vi "Filter For Replacement Terms.vi"(11 "SubVI in":refnum<vi>) -> (3 "Terms[]":refnum<vi>[](array[refnum]))   [LabVIEW 2020, in "Message Maker.lvlib"]
uses:
  Message Maker.lvlib
  <vilib>/Utility/Data Type/NI_Data Type.lvlib
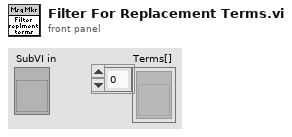
[diagram p1: front panel]
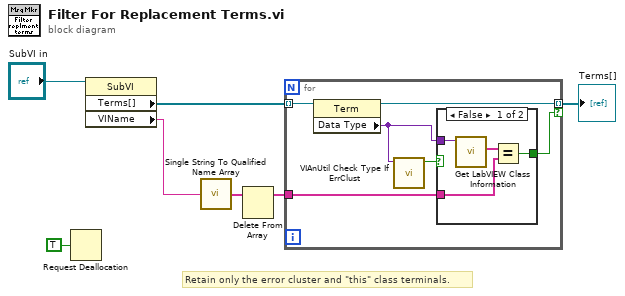
[diagram p0: block diagram]
diagram:
  # "Retain only the error cluster and \"this\" class terminals."
  n1 = Request Deallocation(TRUE ("flag")) -> ()
  n2 = property class="SubVI"(reference="SubVI in") -> ("Terms[]"=w6:refnum<vi>[], "VIName"=w5:string)  [unwired: 1 in, 2 out]
  n3 = call <vilib>:"Single String To Qualified Name Array.vi"("Fully Qualified String"=w5) -> ("Fully Qualified Array"=w4:string[])
  n4 = Delete From Array(array=w4) -> (array with subset deleted=w2:string[])  [unwired: 2 in, 1 out]
  n5 = for {
    tunnel: w6 -> [w13] mode=indexing
    tunnel: [w11] -> w3 mode=indexing if=w10
    tunnel: w2 -> [w8]
    n6 = property class="Term"(reference=w13) -> (reference out=w11:refnum<vi>, "Data Type"=w9:variant)  [unwired: 1 in, 1 out]
    n7 = call <vilib>:"VIAnUtil Check Type If ErrClust.vi"("Data In"=w9) -> ("IsErrClust?"=w12:bool)  [unwired: 9 in, 1 out]
    n8 = case shown="False" w12 {
      selector: w12 -> [_ w18]
      tunnel: [w14 w18] -> w10
      tunnel: w9 -> [w17 _]
      tunnel: w8 -> [w15 _]
      frame False {
        n9 = call <vilib>:"Get LabVIEW Class Information.vi"("variant"=w17) -> ("qualified LabVIEW class name"=w16:string[])  [unwired: 8 in, 2 out]
        n10 = Equal?(x=w16, y=w15) -> (x = y?=w14:bool)
      }
      frame True {
      }
    }
  }
  "Terms[]" <- w3
